vi "Check Moving.vi"(8 "error in (no error)":errorcluster, 11 "Fine SIM Motion Controller in":refnum<class "Fine SIM Motion Controller.lvclass">) -> (0 "error out":errorcluster, 3 "Fine SIM Motion Controller out":refnum<class "Fine SIM Motion Controller.lvclass">)   [LabVIEW 2022 SP3, in "Fine SIM Motion Controller.lvclass"]
uses:
  Fine SIM Motion Controller.lvclass
  C:/Stage-Work/MAS/Axis Objects/Motion Controller/Parent SIM Motion Controller.lvclass
  Motion Controller/Parent SIM Motion Controller.lvclass/Parent SIM Motion Controller.ctl
  Motion Controller/Accessors/Read Sim Axis Data.vi
  Motion Controller/Accessors/Write Sim Axis Data.vi
  Fine SIM Motion Controller.lvclass/Fine SIM Motion Controller.ctl
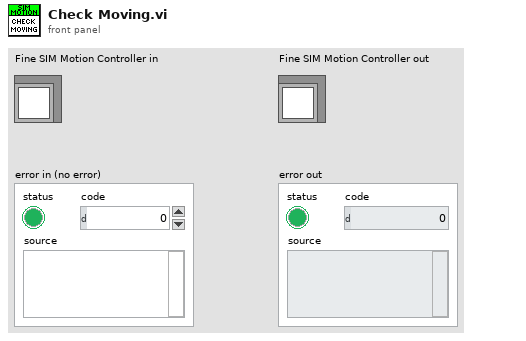
[diagram p1: front panel]
types:
  T1 = typedef "Parent SIM Motion Controller.lvclass/Axis Data.ctl" = cluster{"Axis Parameters":T2, "Axis Settings":T4, "Time Stamp":timestamp}
  T2 = typedef "Parent SIM Motion Controller.lvclass/Axis Parameters.ctl" = cluster{"Moving":bool, "Homed":bool, "Desired Position":dbl, "Current Positon":dbl, "Current Speed":dbl, "Home Status":T3}
  T3 = typedef "Parent SIM Motion Controller.lvclass/Homing Status.ctl" = enum16{"Inital Home Motion", "Final Home Motion", "Done Homing"}
  T4 = typedef "Parent SIM Motion Controller.lvclass/Axis Settings.ctl" = cluster{"Speed":dbl, "Acceleration":dbl}
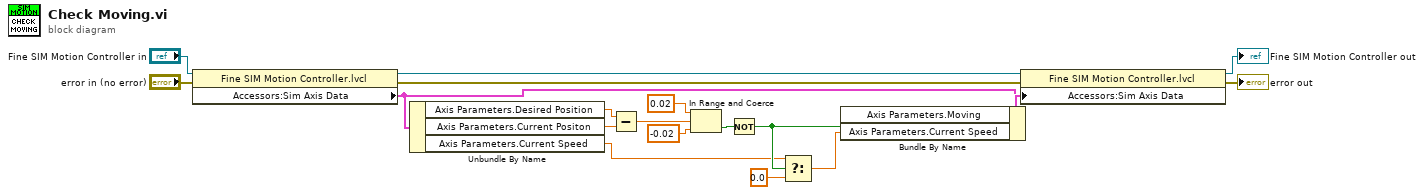
[diagram p0: block diagram]
diagram:
  n1 = property class="Fine SIM Motion Controller.lvcl"(reference="Fine SIM Motion Controller in", error in="error in (no error)") -> (reference out=w8:refnum<class "Fine SIM Motion Controller.lvclass">, error out=w17:errorcluster, "Accessors:Sim Axis Data"=w5:T1)
  n2 = Unbundle By Name(w5) -> ("Axis Parameters.Desired Position"=w10:dbl, "Axis Parameters.Current Positon"=w11:dbl, "Axis Parameters.Current Speed"=w3:dbl)
  n3 = Subtract(x=w10, y=w11) -> (x-y=w12:dbl)
  n4 = In Range and Coerce(upper limit=0.02, x=w12, lower limit=-0.02) -> (In Range?=w15:bool)  [unwired: 1 out]
  n5 = Not(x=w15) -> (.not. x?=w4:bool)
  n6 = Select(t=w3, s=w4, f=0.0) -> (s? t:f=w2:dbl)
  n7 = Bundle By Name(cluster=w5, "Axis Parameters.Moving"=w4, "Axis Parameters.Current Speed"=w2) -> (w6:T1)
  n8 = property class="Fine SIM Motion Controller.lvcl"(reference=w8, error in=w17, "Accessors:Sim Axis Data"=w6) -> (reference out=→"Fine SIM Motion Controller out":refnum<class "Fine SIM Motion Controller.lvclass">, error out=→"error out":errorcluster)
